vi "Protocol Factory_poly.vi"   [LabVIEW 2019]
uses:
  TCP/TCP.lvclass
  UDP/UDP.lvclass
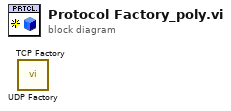
[diagram p0: block diagram]
diagram:
  n1 = call "UDP Factory.vi"() -> ()  [unwired: 10 in, 2 out]
  n2 = call "TCP Factory.vi"() -> ()  [unwired: 10 in, 2 out]
